vi "XOR5 New.vi"() -> ()   [LabVIEW 2014]
panel:
  in  "inputs":T1={"Button 1"=TRUE, "Button 2"=TRUE, "Button 3"=TRUE, "Button 4"=TRUE, "Button 5"=FALSE}
  out "XOR5":bool
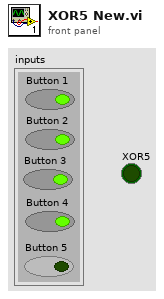
[diagram p1: front panel]
types:
  T1 = cluster{"Button 1":bool, "Button 2":bool, "Button 3":bool, "Button 4":bool, "Button 5":bool}
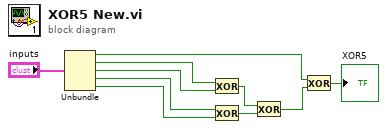
[diagram p0: block diagram]
diagram:
  n1 = Unbundle("inputs") -> ("Button 1"=w5:bool, "Button 2"=w4:bool, "Button 3"=w3:bool, "Button 4"=w2:bool, "Button 5"=w1:bool)
  n2 = Exclusive Or(1:w3, 2:w4) -> (0:w10:bool)
  n3 = Exclusive Or(1:w1, 2:w2) -> (0:w9:bool)
  n4 = Exclusive Or(1:w9, 2:w10) -> (0:w8:bool)
  n5 = Exclusive Or(1:w8, 2:w5) -> (0:→"XOR5":bool)
